vi "stop.vi"(8 "error in (no error)":errorcluster, 11 "WriteSignalsDAQmxPlugin in":refnum<class "SignalWriterDL090202DAQmx.lvclass">) -> (0 "error out":errorcluster, 3 "WriteSignalsDAQmxPlugin out":refnum<class "SignalWriterDL090202DAQmx.lvclass">)   [LabVIEW 2010, in "SignalWriterDL090202DAQmx.lvclass"]
uses:
  SignalWriterDL090202DAQmx.lvclass
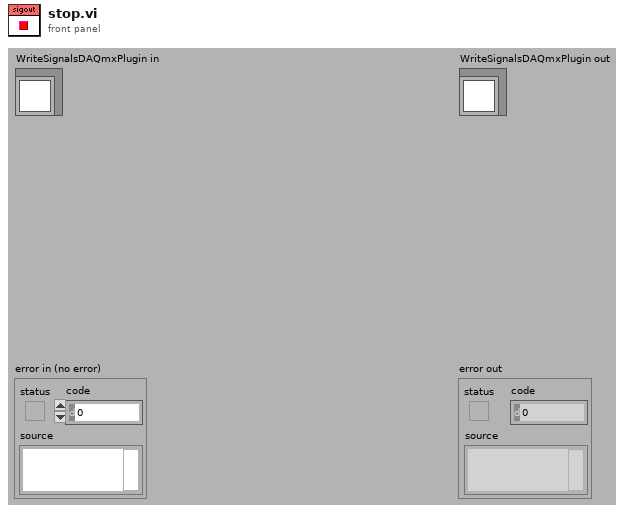
[diagram p1: front panel]
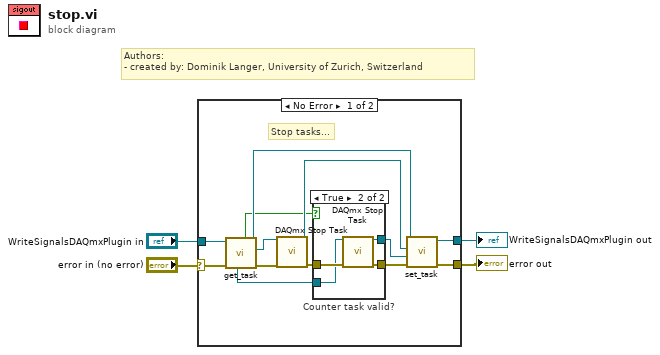
[diagram p0: block diagram]
diagram:
  # "Authors: \n- created by: Dominik Langer, University of Zurich, Switzerland"
  n1 = case shown="No Error" "error in (no error)" {
    selector: "error in (no error)" -> [w17 w25]
    tunnel: [w15 w25] -> w3
    tunnel: [w12 w24] -> w1
    tunnel: "WriteSignalsDAQmxPlugin in" -> [w14 w24]
    frame No Error {
      # "Stop tasks..."
      n2 = call-dynamic "get_task.vi"("error in (no error)"=w17, "DAQmxWriteSignals in"=w14) -> ("error out"=w16:errorcluster, "writer task"=w11:refnum<k21>, "DAQmxWriteSignals out"=w13:refnum<class "SignalWriterDL090202DAQmx.lvclass">, "counter task valid?"=w5:bool, "counter task"=w7:refnum<k21>)  [unwired: 5 out]
      n3 = call <vilib>:"DAQmx Stop Task.vi"("task/channels in"=w11, "error in"=w16) -> ("task out"=w10:refnum<k21>, "error out"=w9:errorcluster)  [unwired: 12 out]
      n4 = case "Counter task valid?" shown="True" w5 {
        tunnel: w9 -> [w19 w23]
        tunnel: [w19 w22] -> w8
        tunnel: w7 -> [w18 w21]
        tunnel: [w18 w20] -> w6
        frame False {
        }
        frame True {
          n5 = call <vilib>:"DAQmx Stop Task.vi"("task/channels in"=w21, "error in"=w23) -> ("task out"=w20:refnum<k21>, "error out"=w22:errorcluster)  [unwired: 12 out]
        }
      }
      n6 = call-dynamic "set_task.vi"("error in (no error)"=w8, "counter task"=w6, "output task"=w10, "DAQmxWriteSignals in"=w13) -> ("error out"=w15:errorcluster, "DAQmxWriteSignals out"=w12:refnum<class "SignalWriterDL090202DAQmx.lvclass">)  [unwired: 6 out]
    }
    frame Error {
    }
  }
  "error out" <- w3
  "WriteSignalsDAQmxPlugin out" <- w1
